vi "RT Loop system status update.vi"(8 "error in (no error)":errorcluster, 11 "system status update interval (ms)":u32=1000 min=500 max=5000) -> ()   [LabVIEW 2016]
uses:
  Message Queue/System notification queue name (constant).ctl
  <vilib>/FPGAPlugInAG/cRIO-9074/niLvFpga_Open_cRIO-9074.vi
  <vilib>/rvi/interface/common/dynamic/niFpgaDynamicAddResources.vi
  Globals/RT Stop.vi
  <vilib>/Utility/error.llb/Error Cluster From Error Code.vi
  <vilib>/rvi/errors/niLvFpgaAdjustHostInterfaceError.vi
  <vilib>/rvi/interface/nirviOpenFPGA/nirviOpenFPGA.xnode
  FPGA Bitfiles/remotecontroller_FPGATarget_FPGAMain_RhGo+c1SRDI.lvbitx
  FPGA Main.vi
  <vilib>/rvi/interface/nirviReadWriteControl/nirviReadWriteControl.xnode
  <vilib>/NI_Real-Time Target Support.lvlib
  <vilib>/nisyscfg/nisyscfg.lvlib
  Message Queue/Message Queue.lvlib
  <resource>/objmgr/nisysapi.rc
  NiFpgaLv.dll
  <vilib>/rvi/interface/Simulation/niFpgaSimulationCallBeginRW.vi
panel:
  out "error out":errorcluster
  out "status summary string":string
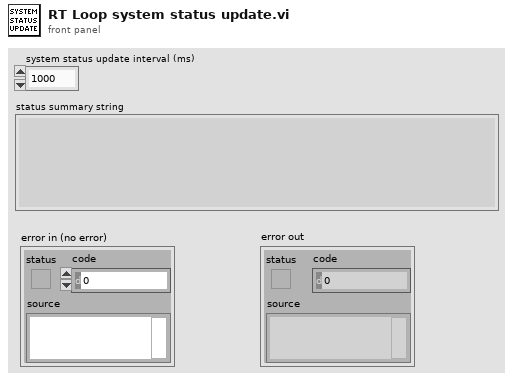
[diagram p1: front panel]
types:
  T1 = typedef "Message Queue.lvlib/System notification queue name (constant).ctl" = string
  T2 = enum16{"Safe State", "I/O with PID Control", "Fast Output Only"}
  T3 = typedef "NI_Real-Time Target Support.lvlib/RT CPU Load.ctl" = cluster{"Total (%)":dbl, "Time Critical (%)":dbl, "Timed Structures (%)":dbl, "High (%)":dbl, "Above Normal (%)":dbl, "Normal (%)":dbl, "Background (%)":dbl, "Idle (%)":dbl, "ISR (%)":dbl}
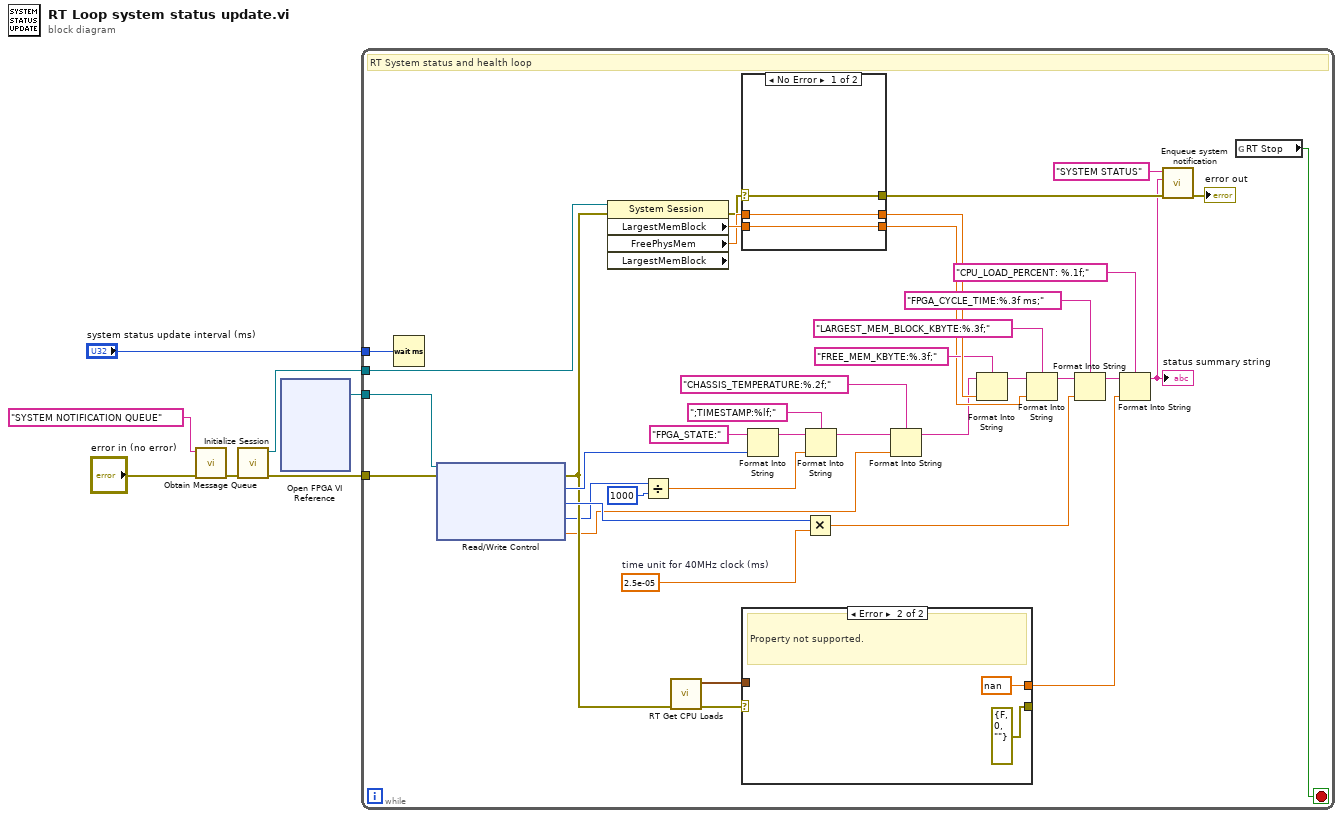
[diagram p0: block diagram]
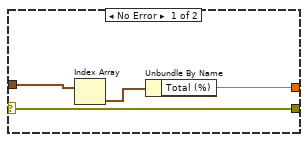
[diagram p2: hidden frame]
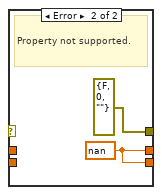
[diagram p3: hidden frame]
diagram:
  n1 = call "Obtain Message Queue.vi"("error in (no error)"="error in (no error)", "name (unnamed)"=T1 "SYSTEM NOTIFICATION QUEUE" ("System notification queue name")) -> ("error out"=w6:errorcluster)  [unwired: 7 in, 2 out]
  n2 = call <vilib>:"Initialize Session.vi"("error in (no error)"=w6) -> ("error out"=w5:errorcluster, "Session out"=w3:refnum<k21>)  [unwired: 9 in]
  n3 = xnode "Open FPGA VI Reference"() -> ("FPGA VI Reference Out"=w4:refnum<k20>)  [unwired: 2 in, 1 out]
  n4 = while {
    tunnel: w5 -> [w46]
    tunnel: w4 -> [w45]
    tunnel: w3 -> [w44]
    tunnel: "system status update interval (ms)" -> [w32]
    stop <- w33 stop-if-true
    w29 = 2.5e-05  # time unit for 40MHz clock (ms)
    # "RT System status and health loop"
    n5 = Wait (ms)(milliseconds to wait=w32) -> ()  [unwired: 1 out]
    n6 = xnode "Read/Write Control"("FPGA VI Reference In"=w45, "error in"=w46) -> ("error out"=w19:errorcluster, "FPGA state"=w40:T2, "ticks"=w30:i64, "time stamp (ms)"=w16:u64, "Chassis Temperature"=w11:sgl)  [unwired: 1 out]
    n7 = property class="System Session" props=["LargestMemBlock", "FreePhysMem", "LargestMemBlock"](reference=w44, error in=w19) -> (error out=w41:errorcluster, "LargestMemBlock"=w43:dbl, "FreePhysMem"=w42:dbl)  [unwired: 2 out]
    n8 = Divide(x=w16, y=u64 1000) -> (x/y=w14:dbl)
    n9 = call <vilib>:"RT Get CPU Loads.vi"("error in (no error)"=w19) -> ("error out"=w20:errorcluster, "CPU loads"=w18:T3[])  [unwired: 9 in]
    n10 = case shown="No Error" w41 {
      selector: w41 -> [w53 _]
      tunnel: w43 -> [w54 _]
      tunnel: [w54 w57] -> w34
      tunnel: w42 -> [w55 _]
      tunnel: [w55 w57] -> w38
      tunnel: [w53 errorcluster {"status"=FALSE, "code"=0, "source"=""} ("error IO")] -> w25
      frame No Error {
      }
      frame Error {
        w57 = nan
        # "Property not supported."
      }
    }
    n11 = case shown="Error" w20 {
      selector: w20 -> [w50 _]
      tunnel: [w47 nan] -> w17
      tunnel: [w50 errorcluster {"status"=FALSE, "code"=0, "source"=""} ("error IO")] -> _
      tunnel: w18 -> [w48 _]
      frame No Error {
        n12 = Index Array(array=w48) -> (element=w49:T3)  [unwired: 1 in]
        n13 = Unbundle By Name(w49) -> ("Total (%)"=w47:dbl)
      }
      frame Error {
        # "Property not supported."
      }
    }
    n14 = Format Into String(initial string="FPGA_STATE:", w40) -> (resulting string=w12:string)  [unwired: 2 in, 1 out]
    n15 = Multiply(x=w30, y=w29) -> (x*y=w28:dbl)
    n16 = Format Into String(format string=";TIMESTAMP:%lf;", initial string=w12, w14) -> (resulting string=w9:string)  [unwired: 1 in, 1 out]
    n17 = Format Into String(format string="CHASSIS_TEMPERATURE:%.2f;", initial string=w9, w11) -> (resulting string=w8:string)  [unwired: 1 in, 1 out]
    n18 = Format Into String(format string="FREE_MEM_KBYTE:%.3f;", initial string=w8, w38) -> (resulting string=w36:string)  [unwired: 1 in, 1 out]
    n19 = Format Into String(format string="LARGEST_MEM_BLOCK_KBYTE:%.3f;", initial string=w36, w34) -> (resulting string=w31:string)  [unwired: 1 in, 1 out]
    n20 = Format Into String(format string="FPGA_CYCLE_TIME:%.3f ms;", initial string=w31, w28) -> (resulting string=w23:string)  [unwired: 1 in, 1 out]
    n21 = Format Into String(format string="CPU_LOAD_PERCENT: %.1f;", initial string=w23, w17) -> (resulting string=w22:string)  [unwired: 1 in, 1 out]
    "status summary string" <- w22
    n22 = call "Enqueue system notification.vi"("error in (no error)"=w25, "Message Data"=w22, "system message"="SYSTEM STATUS" ("message")) -> ("error out"=→"error out":errorcluster)  [unwired: 8 in]
    n23 = global read "RT Stop.vi" "RT Stop"() -> (w33:bool)
  }
